vi "CRYGroup Manipulate Sub.vi"(5 "Type":enum16{"Curves", "Values", "Results", "WFM"}(ring), 7 "sAction":string, 8 "sOption":string, 9 "nData":i32[](array[numeric]), 10 "sData":string[](array[string]), 11 "Tree in":refnum<vi>) -> (0 "bData out":bool, 1 "Step&Tags Out":T1(array[cluster]), 2 "nData Out":i32[](array[numeric]), 3 "Tree Out":refnum<vi>, 4 "sData Out":string[](array[string]))   [LabVIEW 2013]
uses:
  CRYProject/CRYProject Editor Global.vi
  Global/CRYCurve Library Global.vi
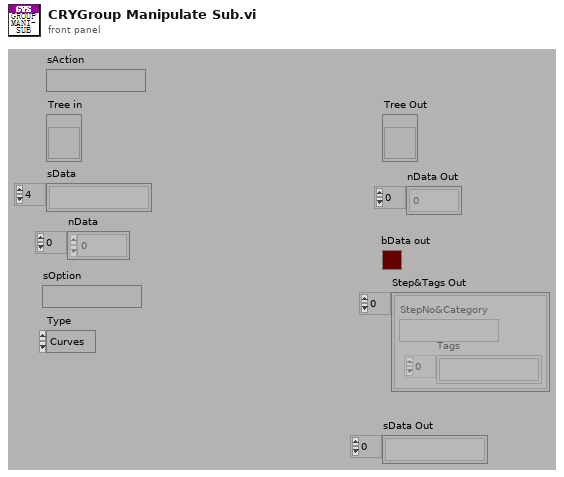
[diagram p1: front panel]
types:
  T1 = cluster{"Tags":string[], "StepNo&Category":string}[]
  T2 = cluster{"Tags":string[], "StepNo&Category":string}
  T3 = typedef "CRYStep.ctl" = cluster{"No.VI":i32, "Category":string, "StepName":string, "Seq setup flattened":string, "Comment":string, "Steps config.":bool[], "Jump config":i32[], "Start":dbl, "Increment":dbl, "Name":string, "Unit":string, "Y data":u16, "Y prefix":string, "Y dB ref":dbl, "Y unit":string, "Repeat State Array":cluster{"Start":dbl, "Increment":dbl, "Count":i32, "Num":i32}[]}
  T4 = typedef "CRYData Cluster.ctl" = cluster{"Name":string, "Curve":cluster{"x":dbl, "y":dbl, "z":dbl}[], "X data":u16, "Y data":u16, "Z data":u16, "X axis":u16, "Y axis":u16, "Z axis":u16, "X unit":string, "Y unit":string, "Z unit":string, "X dB ref":dbl, "Y dB ref":dbl, "Z dB ref":dbl, "single val":bool, "protected":bool, "display X":bool, "display Y":bool, "display Z":bool, "Test Info":string, "Step No.":i32, "Plot Settings":cluster{"Color":u32, "Interpolation":u8, "Point Style":u8, "Line Style":u8, "Point Color":u32, "Line Width":u8, "Bar Plot Style":u8, "Fill To":i16}, "AutoProtect":bool}
  T5 = typedef "CRYWaveform Cluster.ctl" = cluster{"Waveform":cluster{"X0":dbl, "dX":dbl, "Y":sgl[]}, "X data":u16, "Y data":u16, "Y axis":u16, "X unit":string, "Y unit":string, "Y dB ref":dbl, "display Y":bool, "display X":bool, "Overload?":bool, "Test Info":string, "Step No.":i32, "Name":string, "protected":bool, "Sqc history":string[], "Signal Channel ID":i32, "Plot Settings":cluster{"Color":u32, "Interpolation":u8, "Point Style":u8, "Line Style":u8, "Point Color":u32, "Line Width":u8, "Bar Plot Style":u8, "Fill To":i16}, "AutoProtect":bool}
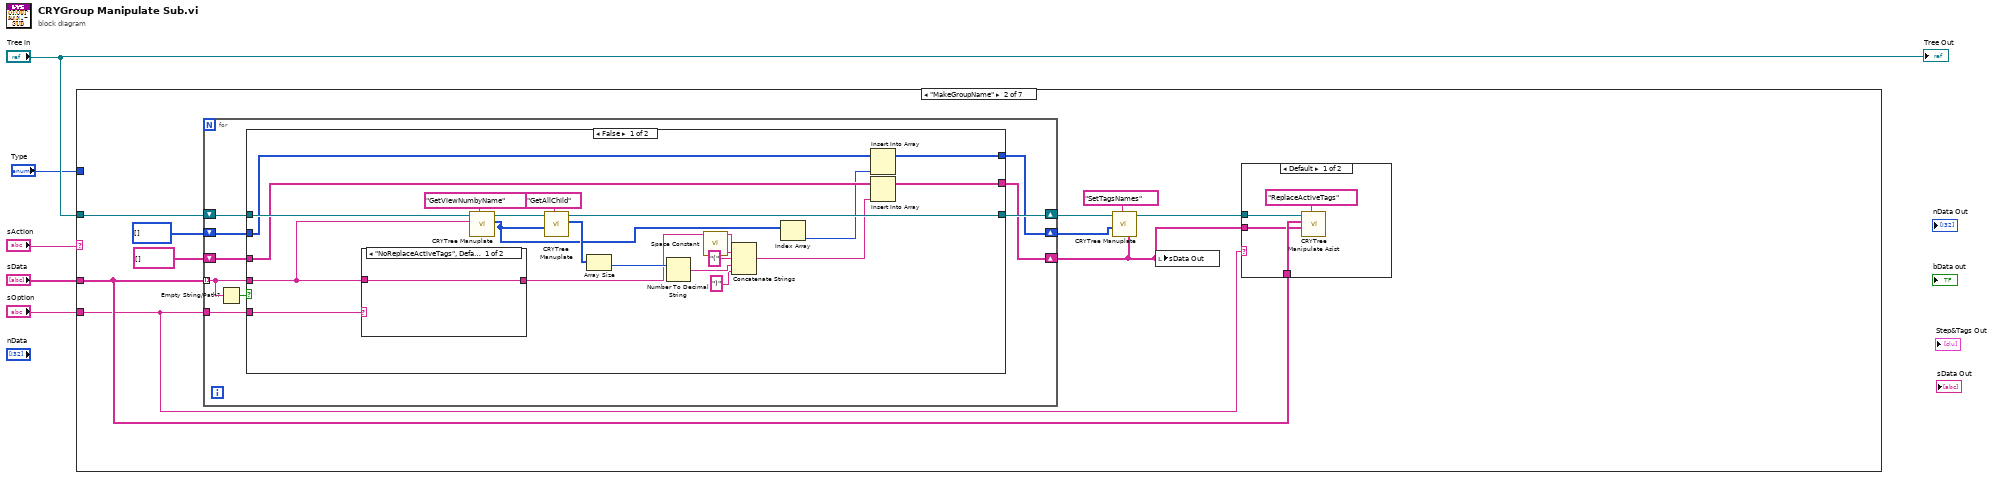
[diagram p0: block diagram]
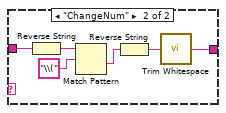
[diagram p4: hidden frame]
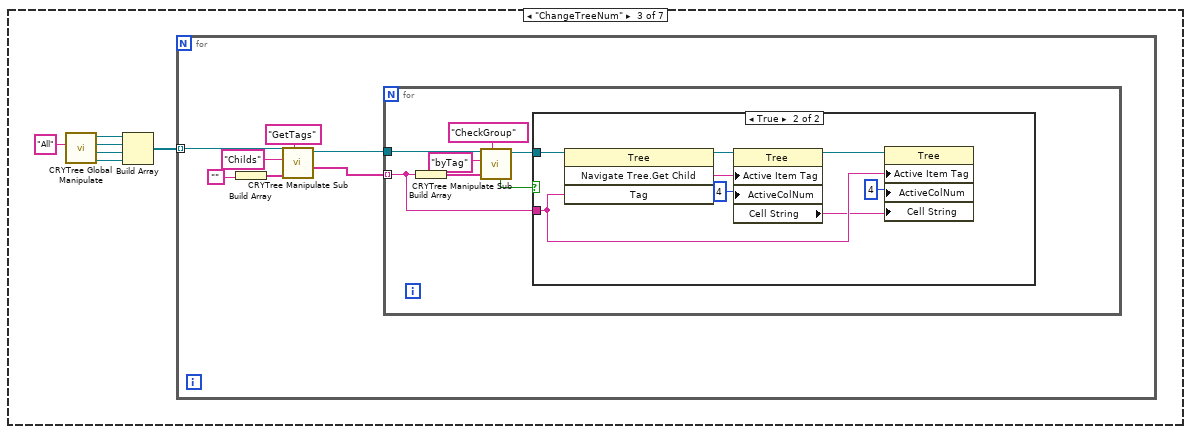
[diagram p6: hidden frame]
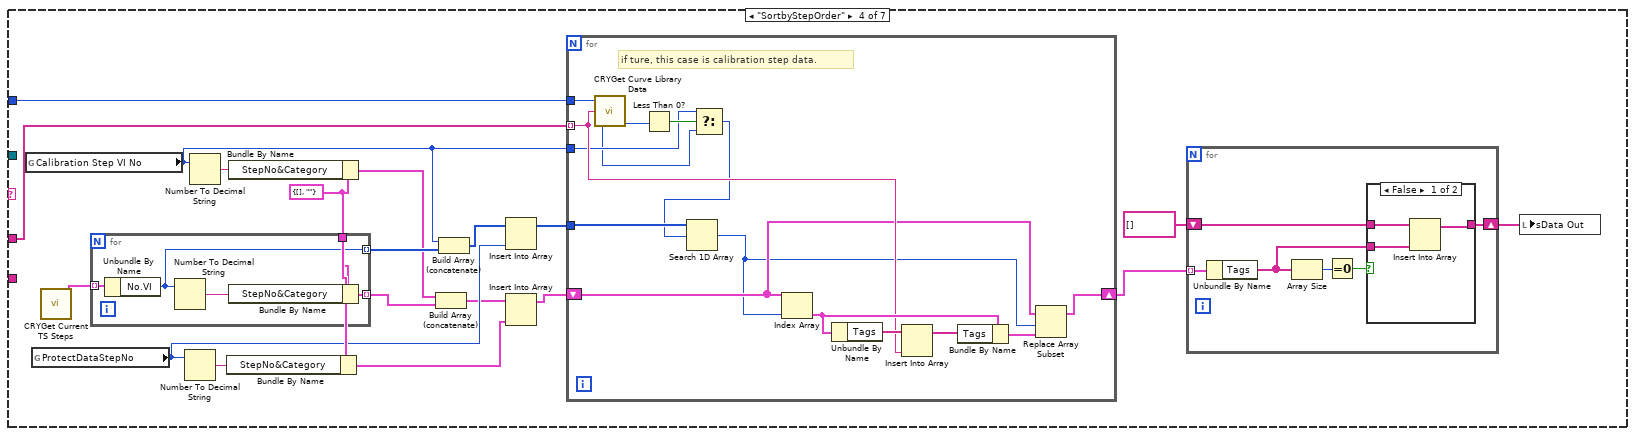
[diagram p8: hidden frame]
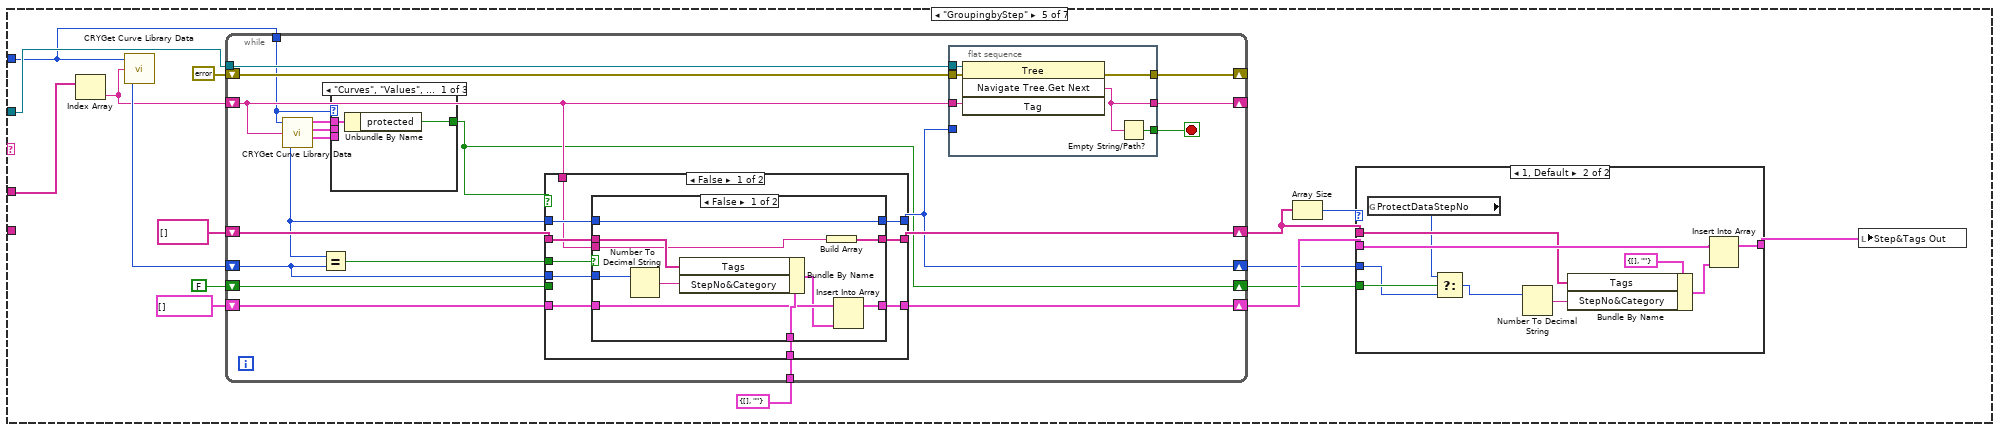
[diagram p10: hidden frame]
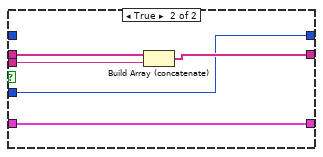
[diagram p12: hidden frame]
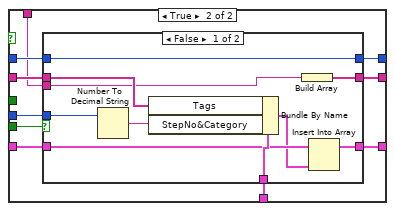
[diagram p13: hidden frame]
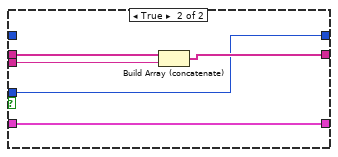
[diagram p14: hidden frame]
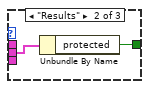
[diagram p15: hidden frame]
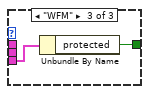
[diagram p16: hidden frame]
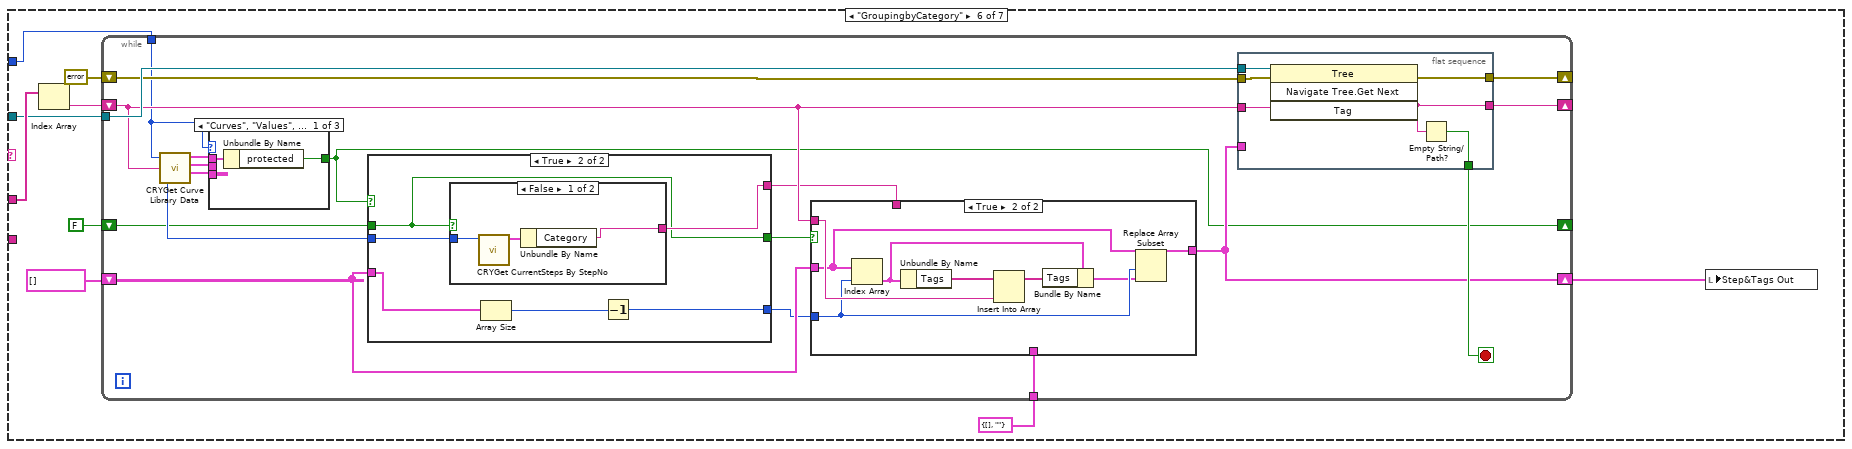
[diagram p17: hidden frame]
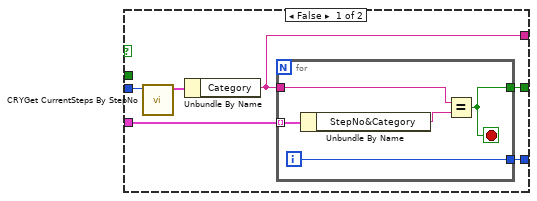
[diagram p18: hidden frame]
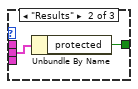
[diagram p20: hidden frame]
diagram:
  n1 = case shown="\"MakeGroupName\"" "sAction" {
    tunnel: "Tree in" -> [_ w15 _ _ w147 w252 w325]
    tunnel: "sData" -> [_ w11 _ w104 w152 w255 w324]
    tunnel: "sOption" -> [_ w6 _ _ _ _ _]
    tunnel: "Type" -> [_ _ _ w105 w146 w251 _]
    frame Default {
    }
    frame "MakeGroupName" {
      n2 = for {
        tunnel: w11 -> [w26] mode=indexing
        tunnel: w6 -> [w25]
        shift-right: [w24] -> w13
        shift-left: w15 -> [w28]
        shift-right: [w21] -> w8
        shift-left: i32[] [] -> [w23]
        shift-right: [w20] -> w7
        shift-left: string[] [] -> [w22]
        n3 = Empty String/Path?(string/path=w26) -> (empty?=w27:bool)
        n4 = case shown="False" w27 {
          tunnel: w28 -> [w40 w59]
          tunnel: w26 -> [w38 _]
          tunnel: w25 -> [w39 _]
          tunnel: [w35 w59] -> w24
          tunnel: w23 -> [w34 w58]
          tunnel: w22 -> [w33 w57]
          tunnel: [w30 w58] -> w21
          tunnel: [w29 w57] -> w20
          frame False {
            n5 = case shown="\"NoReplaceActiveTags\", Default" w39 {
              tunnel: w38 -> [w50 w52]
              tunnel: [w50 w51] -> w37
              frame "NoReplaceActiveTags", Default {
              }
              frame "ChangeNum" {
                n6 = Reverse String(1:w52) -> (0:w56:string)
                n7 = Match Pattern(string=w56, regular expression="\\(" ("search string/char (-)")) -> (after substring=w54:string)  [unwired: 1 in, 3 out]
                n8 = Reverse String(1:w54) -> (0:w53:string)
                n9 = call <vilib>:"Trim Whitespace.vi"("string"=w53) -> ("trimmed string"=w51:string)  [unwired: 1 in]
              }
            }
            n10 = call "CRYTree Manuplate.vi"("sAction"="GetViewNumbyName", "sOption"=w38, "Tree in"=w40) -> ("nData Out"=w36:i32[], "Tree Out"=w45:refnum<vi>)  [unwired: 5 in, 2 out]
            n11 = call "CRYTree Manuplate.vi"("sAction"="GetAllChild", "nData"=w36, "Tree in"=w45) -> ("nData Out"=w48:i32[], "Tree Out"=w35:refnum<vi>)  [unwired: 5 in, 2 out]
            n12 = Array Size(array=w48) -> (size(s)=w47:i32)
            n13 = Number To Decimal String(number=w47) -> (decimal integer string=w43:string)  [unwired: 1 in]
            n14 = call <vilib>:"Space Constant.vi"() -> ("String"=w41:string)
            n15 = Concatenate Strings(w37, w41, "(" ("string"), w43, ")" ("string")) -> (w32:string)
            n16 = Index Array(array=w36) -> (element=w31:i32)  [unwired: 1 in]
            n17 = Insert Into Array(array=w34, new element=w31) -> (w30:i32[])  [unwired: 1 in]
            n18 = Insert Into Array(array=w33, new element=w32) -> (w29:string[])  [unwired: 1 in]
          }
          frame True {
          }
        }
      }
      n19 = call "CRYTree Manuplate.vi"("sData"=w7, "sAction"="SetTagsNames", "nData"=w8, "Tree in"=w13) -> ("Tree Out"=w12:refnum<vi>)  [unwired: 4 in, 3 out]
      n20 = local write "sData Out"(w7) -> ()
      n21 = case shown="Default" w6 {
        tunnel: w12 -> [w18 _]
        tunnel: w11 -> [w17 _]
        tunnel: w7 -> [w16 _]
        frame Default {
          n22 = call "CRYTree Manipulate Asist.vi"("sAction"="ReplaceActiveTags", "sNewTags"=w16, "sOrgTags"=w17, "Tree in"=w18) -> ()  [unwired: 5 in, 3 out]
        }
        frame "NoReplaceActiveTags" {
        }
      }
    }
    frame "ChangeTreeNum" {
      n23 = call "CRYTree Global Manipulate.vi"("sOption"="All") -> ("WFM Tree"=w61:refnum<vi>, "Results Tree"=w62:refnum<vi>, "Values Tree"=w63:refnum<vi>, "Tree/Curve Tree"=w64:refnum<vi>)  [unwired: 7 in]
      n24 = Build Array(w64, w63, w62, w61) -> (w60:refnum<vi>[])
      n25 = for {
        tunnel: w60 -> [w66] mode=indexing
        n26 = Build Array("") -> (w70:string[])
        n27 = call "CRYTree Manipulate Sub.vi"("sAction"="GetTags", "sData"=w70, "sOption"="Childs", "Tree in"=w66) -> ("sData Out"=w67:string[], "Tree Out"=w68:refnum<vi>)  [unwired: 3 in, 3 out]
        n28 = for {
          tunnel: w67 -> [w74] mode=indexing
          tunnel: w68 -> [w76]
          n29 = Build Array(w74) -> (w77:string[])
          n30 = call "CRYTree Manipulate Sub.vi"("sAction"="CheckGroup", "sData"=w77, "sOption"="byTag", "Tree in"=w76) -> ("Tree Out"=w73:refnum<vi>, "bCategory"=w75:bool)  [unwired: 3 in, 3 out]
          n31 = case shown="True" w75 {
            tunnel: w74 -> [_ w83]
            tunnel: w73 -> [_ w87]
            frame False {
            }
            frame True {
              n32 = invoke class="Tree" method="Navigate Tree.Get Child"(reference=w87, "Tag"=w83) -> (reference out=w86:refnum<vi>, "Navigate Tree:Get Child"=w85:string)  [unwired: 2 in, 2 out]
              n33 = property class="Tree"(reference=w86, "Active Item Tag"=w85, "ActiveColNum"=4 ("Active Cell:Active Column Number")) -> (reference out=w80:refnum<vi>, "Cell String"=w81:string)  [unwired: 1 in, 1 out]
              n34 = property class="Tree"(reference=w80, "Active Item Tag"=w83, "ActiveColNum"=4 ("Active Cell:Active Column Number"), "Cell String"=w81) -> ()  [unwired: 1 in, 2 out]
            }
          }
        }
      }
    }
    frame "SortbyStepOrder" {
      w99 = T2 {"Tags"=[], "StepNo&Category"=""} ("Cluster")
      n35 = global read "CRYProject Editor Global.vi" "Calibration Step VI No"() -> (w92:i32)
      n36 = global read "CRYCurve Library Global.vi" "ProtectDataStepNo"() -> (w94:i32)
      n37 = call "CRYGet Current TS Steps.vi"() -> ("Steps"=w106:T3[])  [unwired: 7 in, 4 out]
      n38 = for {
        tunnel: w106 -> [w136] mode=indexing
        tunnel: [w134] -> w89 mode=indexing
        tunnel: w99 -> [w133]
        tunnel: [w132] -> w93 mode=indexing
        n39 = Unbundle By Name(w136) -> ("No.VI"=w132:i32)
        n40 = Number To Decimal String(number=w132) -> (decimal integer string=w135:string)  [unwired: 1 in]
        n41 = Bundle By Name(cluster=w133, "StepNo&Category"=w135) -> (w134:T2)
      }
      n42 = Number To Decimal String(number=w94) -> (decimal integer string=w95:string)  [unwired: 1 in]
      n43 = Number To Decimal String(number=w92) -> (decimal integer string=w100:string)  [unwired: 1 in]
      n44 = Bundle By Name(cluster=w99, "StepNo&Category"=w95) -> (w96:T2)
      n45 = Bundle By Name(cluster=w99, "StepNo&Category"=w100) -> (w90:T2)
      n46 = Build Array (concatenate)(w90, w89) -> (w88:T1)
      n47 = Build Array (concatenate)(w92, w93) -> (w91:i32[])
      n48 = Insert Into Array(array=w91, new element=w94) -> (w98:i32[])  [unwired: 1 in]
      n49 = Insert Into Array(array=w88, new element=w96) -> (w97:T1)  [unwired: 1 in]
      n50 = for {
        tunnel: w105 -> [w131]
        tunnel: w104 -> [w126] mode=indexing
        tunnel: w98 -> [w130]
        shift-right: [w123] -> w103
        shift-left: w97 -> [w125]
        tunnel: w92 -> [w120]
        # "if ture, this case is calibration step data."
        n51 = call "CRYGet Curve Library Data.vi"("Type"=w131, "Data Name"=w126) -> ("Step No."=w119:i32, "index"=w122:i32)  [unwired: 3 out]
        n52 = Less Than 0?(x=w122) -> (x < 0?=w121:bool)
        n53 = Select(t=w120, s=w121, f=w119) -> (s? t:f=w118:i32)
        n54 = Search 1D Array(1D array=w130, element=w118) -> (index of element=w117:i32)  [unwired: 1 in]
        n55 = Index Array(array=w125, index=w117) -> (element=w128:T2)
        n56 = Unbundle By Name(w128) -> ("Tags"=w129:string[])
        n57 = Insert Into Array(array=w129, new element=w126) -> (w127:string[])  [unwired: 1 in]
        n58 = Bundle By Name(cluster=w128, "Tags"=w127) -> (w124:T2)
        n59 = Replace Array Subset(array=w125, new element=w124, index=w117) -> (w123:T1)
      }
      n60 = for {
        tunnel: w103 -> [w112] mode=indexing
        shift-right: [w109] -> w101
        shift-left: string[] [] ("Tags") -> [w110]
        n61 = Unbundle By Name(w112) -> ("Tags"=w107:string[])
        n62 = Array Size(array=w107) -> (size(s)=w111:i32)
        n63 = Equal To 0?(x=w111) -> (x = 0?=w108:bool)
        n64 = case shown="False" w108 {
          tunnel: w110 -> [w115 w116]
          tunnel: [w114 w116] -> w109
          tunnel: w107 -> [w113 _]
          frame False {
            n65 = Insert Into Array(array=w115, new element=w113) -> (w114:string[])  [unwired: 1 in]
          }
          frame True {
          }
        }
      }
      n66 = local write "sData Out"(w101) -> ()
    }
    frame "GroupingbyStep" {
      n67 = Index Array(array=w152) -> (element=w149:string)  [unwired: 1 in]
      n68 = call "CRYGet Curve Library Data.vi"("Type"=w146, "Data Name"=w149) -> ("Step No."=w150:i32)  [unwired: 4 out]
      n69 = while {
        tunnel: w147 -> [w184]
        shift-right: [w173] -> _
        shift-left: w149 -> [w170]
        shift-right: [w182] -> _
        shift-left: errorcluster {"status"=FALSE, "code"=0, "source"=""} ("error out") -> [w183]
        shift-right: [w181] -> w137
        shift-left: string[] [] -> [w180]
        tunnel: w146 -> [w169]
        shift-right: [w172] -> w143
        shift-left: w150 -> [w179]
        tunnel: T2 {"Tags"=[], "StepNo&Category"=""} ("Cluster") -> [w177]
        shift-right: [w175] -> w145
        shift-left: T1 [] ("Array") -> [w176]
        shift-right: [w164] -> w138
        shift-left: FALSE ("x = y?") -> [w165]
        stop <- w178 stop-if-true
        n70 = call "CRYGet Curve Library Data.vi"("Type"=w169, "Data Name"=w170) -> ("Step No."=w174:i32, "Curve"=w168:T4, "Value"=w167:T4, "Wave"=w166:T5)  [unwired: 1 out]
        n71 = Equal?(x=w174, y=w179) -> (x = y?=w171:bool)
        n72 = case shown="\"Curves\", \"Values\", Default" w169 {
          tunnel: w168 -> [w236 _ _]
          tunnel: w167 -> [_ w237 _]
          tunnel: w166 -> [_ _ w239]
          tunnel: [w235 w238 w240] -> w164
          frame "Curves", "Values", Default {
            n73 = Unbundle By Name(w236) -> ("protected"=w235:bool)
          }
          frame "Results" {
            n74 = Unbundle By Name(w237) -> ("protected"=w238:bool)
          }
          frame "WFM" {
            n75 = Unbundle By Name(w239) -> ("protected"=w240:bool)
          }
        }
        n76 = case shown="False" w164 {
          tunnel: [w194 w219] -> w181
          tunnel: w180 -> [w193 w218]
          tunnel: w179 -> [w192 w217]
          tunnel: w177 -> [w191 w216]
          tunnel: w176 -> [w190 w215]
          tunnel: [w189 w214] -> w175
          tunnel: w174 -> [w188 w213]
          tunnel: [w187 w212] -> w172
          tunnel: w171 -> [w186 _]
          tunnel: w170 -> [w185 w211]
          tunnel: w165 -> [_ w210]
          frame False {
            n77 = case shown="False" w186 {
              tunnel: w193 -> [w203 w209]
              tunnel: [w197 w208] -> w194
              tunnel: w185 -> [w198 w207]
              tunnel: w191 -> [w204 _]
              tunnel: w192 -> [w196 w206]
              tunnel: w190 -> [w202 w205]
              tunnel: [w200 w205] -> w189
              tunnel: w188 -> [w199 _]
              tunnel: [w199 w206] -> w187
              frame False {
                n78 = Number To Decimal String(number=w196) -> (decimal integer string=w195:string)  [unwired: 1 in]
                n79 = Bundle By Name(cluster=w204, "Tags"=w203, "StepNo&Category"=w195) -> (w201:T2)
                n80 = Build Array(w198) -> (w197:string[])
                n81 = Insert Into Array(array=w202, new element=w201) -> (w200:T1)  [unwired: 1 in]
              }
              frame True {
                n82 = Build Array (concatenate)(w209, w207) -> (w208:string[])
              }
            }
          }
          frame True {
            n83 = case shown="False" w210 {
              tunnel: w218 -> [w228 w234]
              tunnel: [w222 w233] -> w219
              tunnel: w211 -> [w223 w232]
              tunnel: w216 -> [w229 _]
              tunnel: w217 -> [w220 w231]
              tunnel: w215 -> [w227 w230]
              tunnel: [w225 w230] -> w214
              tunnel: w213 -> [w224 _]
              tunnel: [w224 w231] -> w212
              frame False {
                n84 = Number To Decimal String(number=w220) -> (decimal integer string=w221:string)  [unwired: 1 in]
                n85 = Bundle By Name(cluster=w229, "Tags"=w228, "StepNo&Category"=w221) -> (w226:T2)
                n86 = Build Array(w223) -> (w222:string[])
                n87 = Insert Into Array(array=w227, new element=w226) -> (w225:T1)  [unwired: 1 in]
              }
              frame True {
                n88 = Build Array (concatenate)(w234, w232) -> (w233:string[])
              }
            }
          }
        }
        n89 = flat-sequence {
          tunnel: w184 -> [w246]
          tunnel: w183 -> [w245]
          tunnel: [w244] -> w182
          tunnel: [w243] -> w178
          tunnel: [w242] -> w173
          tunnel: w170 -> [w241]
          tunnel: w172 -> [_]
          frame #0 {
            n90 = invoke class="Tree" method="Navigate Tree.Get Next"(reference=w246, error in=w245, "Tag"=w241) -> (error out=w244:errorcluster, "Navigate Tree:Get Next Item"=w242:string)  [unwired: 1 in, 2 out]
            n91 = Empty String/Path?(string/path=w242) -> (empty?=w243:bool)
          }
        }
      }
      n92 = Array Size(array=w137) -> (size(s)=w142:i32)
      n93 = case shown="1, Default" w142 {
        tunnel: w145 -> [w153 w163]
        tunnel: [w153 w161] -> w144
        tunnel: w143 -> [_ w156]
        tunnel: w138 -> [_ w157]
        tunnel: w137 -> [_ w158]
        frame 0 {
        }
        frame 1, Default {
          n94 = global read "CRYCurve Library Global.vi" "ProtectDataStepNo"() -> (w154:i32)
          n95 = Select(t=w154, s=w157, f=w156) -> (s? t:f=w155:i32)
          n96 = Number To Decimal String(number=w155) -> (decimal integer string=w159:string)  [unwired: 1 in]
          n97 = Bundle By Name(cluster=T2 {"Tags"=[], "StepNo&Category"=""} ("Cluster"), "Tags"=w158, "StepNo&Category"=w159) -> (w162:T2)
          n98 = Insert Into Array(array=w163, new element=w162) -> (w161:T1)  [unwired: 1 in]
        }
      }
      n99 = local write "Step&Tags Out"(w144) -> ()
    }
    frame "GroupingbyCategory" {
      n100 = Index Array(array=w255) -> (element=w253:string)  [unwired: 1 in]
      n101 = while {
        tunnel: w252 -> [w273]
        shift-right: [w265] -> _
        shift-left: w253 -> [w268]
        shift-right: [w263] -> _
        shift-left: errorcluster {"status"=FALSE, "code"=0, "source"=""} ("error out") -> [w264]
        tunnel: w251 -> [w261]
        tunnel: T2 {"Tags"=[], "StepNo&Category"=""} ("Cluster") -> [w267]
        shift-right: [w262] -> w248
        shift-left: T1 [] ("Array") -> [w270]
        shift-right: [w256] -> _
        shift-left: FALSE ("protected") -> [w257]
        stop <- w272 stop-if-true
        n102 = call "CRYGet Curve Library Data.vi"("Type"=w261, "Data Name"=w268) -> ("Step No."=w274:i32, "Curve"=w260:T4, "Value"=w259:T4, "Wave"=w258:T5)  [unwired: 1 out]
        n103 = case shown="\"Curves\", \"Values\", Default" w261 {
          tunnel: w260 -> [w296 _ _]
          tunnel: w259 -> [_ w297 _]
          tunnel: w258 -> [_ _ w299]
          tunnel: [w295 w298 w300] -> w256
          frame "Curves", "Values", Default {
            n104 = Unbundle By Name(w296) -> ("protected"=w295:bool)
          }
          frame "Results" {
            n105 = Unbundle By Name(w297) -> ("protected"=w298:bool)
          }
          frame "WFM" {
            n106 = Unbundle By Name(w299) -> ("protected"=w300:bool)
          }
        }
        n107 = case shown="True" w256 {
          tunnel: w274 -> [w279 w289]
          tunnel: [w278 w290] -> w271
          tunnel: w270 -> [w277 w288]
          tunnel: [w276 w286] -> w269
          tunnel: [w275 w291] -> w266
          tunnel: w257 -> [_ w290]
          frame False {
            n108 = call "CRYGet CurrentSteps By StepNo.vi"("Step Setup VI No"=w279) -> ("Step"=w280:T3)  [unwired: 8 in, 2 out]
            n109 = Unbundle By Name(w280) -> ("Category"=w275:string)
            n110 = for {
              tunnel: w277 -> [w283] mode=indexing
              tunnel: w275 -> [w284]
              tunnel: [w282] -> w278
              tunnel: [w281] -> w276
              i -> [w281]
              stop <- w282 stop-if-true
              n111 = Unbundle By Name(w283) -> ("StepNo&Category"=w285:string)
              n112 = Equal?(x=w284, y=w285) -> (x = y?=w282:bool)
            }
          }
          frame True {
            n113 = case shown="False" w290 {
              tunnel: [w292 _] -> w291
              tunnel: w289 -> [w293 _]
              frame False {
                n114 = call "CRYGet CurrentSteps By StepNo.vi"("Step Setup VI No"=w293) -> ("Step"=w294:T3)  [unwired: 8 in, 2 out]
                n115 = Unbundle By Name(w294) -> ("Category"=w292:string)
              }
              frame True {
              }
            }
            n116 = Array Size(array=w288) -> (size(s)=w287:i32)
            n117 = Decrement(x=w287) -> (x-1=w286:i32)
          }
        }
        n118 = case shown="True" w271 {
          tunnel: w270 -> [w307 w311]
          tunnel: w269 -> [_ w310]
          tunnel: w268 -> [w303 w312]
          tunnel: [w306 w308] -> w262
          tunnel: w267 -> [w305 _]
          tunnel: w266 -> [w301 _]
          frame False {
            n119 = Build Array(w303) -> (w302:string[])
            n120 = Bundle By Name(cluster=w305, "StepNo&Category"=w301, "Tags"=w302) -> (w304:T2)
            n121 = Insert Into Array(array=w307, new element=w304) -> (w306:T1)  [unwired: 1 in]
          }
          frame True {
            n122 = Index Array(array=w311, index=w310) -> (element=w315:T2)
            n123 = Unbundle By Name(w315) -> ("Tags"=w314:string[])
            n124 = Insert Into Array(array=w314, new element=w312) -> (w313:string[])  [unwired: 1 in]
            n125 = Bundle By Name(cluster=w315, "Tags"=w313) -> (w309:T2)
            n126 = Replace Array Subset(array=w311, new element=w309, index=w310) -> (w308:T1)
          }
        }
        n127 = flat-sequence {
          tunnel: w273 -> [w321]
          tunnel: w268 -> [w320]
          tunnel: [w319] -> w272
          tunnel: [w318] -> w265
          tunnel: w264 -> [w317]
          tunnel: [w316] -> w263
          tunnel: w262 -> [_]
          frame #0 {
            n128 = invoke class="Tree" method="Navigate Tree.Get Next"(reference=w321, error in=w317, "Tag"=w320) -> (error out=w316:errorcluster, "Navigate Tree:Get Next Item"=w318:string)  [unwired: 1 in, 2 out]
            n129 = Empty String/Path?(string/path=w318) -> (empty?=w319:bool)
          }
        }
      }
      n130 = local write "Step&Tags Out"(w248) -> ()
    }
    frame "DeleteEmptyGroup" {
      n131 = flat-sequence {
        tunnel: w325 -> [w329]
        tunnel: w324 -> [w328]
        tunnel: [w329] -> w323
        tunnel: [w326] -> w322
        tunnel: w323 -> [w347]
        tunnel: w322 -> [w346]
        frame #0 {
          n132 = for {
            tunnel: w329 -> [w337]
            tunnel: w328 -> [w333] mode=indexing
            shift-right: [w330] -> w326
            shift-left: string[] [] ("sData") -> [w331]
            n133 = Build Array(w333) -> (w336:string[])
            n134 = call "CRYTree Manipulate Sub.vi"("sAction"="GetTags", "sData"=w336, "sOption"="Childs", "Tree in"=w337) -> ("sData Out"=w335:string[], "Tree Out"=w334:refnum<vi>)  [unwired: 3 in, 3 out]
            n135 = Array Size(array=w335) -> (size(s)=w332:i32)
            n136 = case shown="0" w332 {
              tunnel: w334 -> [w344 _]
              tunnel: w333 -> [w340 _]
              tunnel: w331 -> [w342 w345]
              tunnel: [w341 w345] -> w330
              frame 0 {
                n137 = invoke class="Tree" method="Edit Tree Items.Delete"(reference=w344, "tag"=w340, "Delete Children"=TRUE ("Delete Children?")) -> ()  [unwired: 2 in, 5 out]
                n138 = Insert Into Array(array=w342, new element=w340) -> (w341:string[])  [unwired: 1 in]
              }
              frame 1, Default {
              }
            }
          }
        }
        frame #1 {
          n139 = call "CRYTree Manipulate Asist.vi"("sAction"="RemoveActiveTags", "sOrgTags"=w346, "Tree in"=w347) -> ()  [unwired: 6 in, 3 out]
        }
      }
    }
  }
  "Tree Out" <- "Tree in"
